vi "Kalibrationsprogramm_kapazitiv_yokogawaneu_2550.vi"(2 "Delay [ms]":u32=5000, 3 "Messzeit [ms]":u32=7000, 4 "B-Feld":dbl=5.0, 5 "error in (no error)":errorcluster, 6 "Startwert (V)":dbl=-5.0 min=-30.0 max=30.0 step=0.01, 7 "Stepsize (V)":dbl=1.0 min=0.0, 8 "Endwert (V)":dbl=4.0 min=-25.0 max=25.0 step=0.01) -> (15 "Ausgabe-Cluster":T1={" I (A)"=-5.009899999999962e-06, "Voltage"=42.05182, "B-Feld"=5.0, "Timestamp"=3396872323.6577854} {"Timestamp" format="%#_6f"}, 19 "error out":errorcluster)   [LabVIEW 2009]
uses:
  Instance           2 16Saved   Yokogawa .vi
  <vilib>/Utility/file.llb/Write To Spreadsheet File (DBL).vi
panel:
  out "XY Graph":cluster{dbl[], dbl[]}(graph)={[-5.004999999999957e-06, -3.989950000000041e-06, -2.990100500000007e-06, -1.999999999999981e-06, -9.9000000000001e-07, 2.2830184906463564e-22, 1.0000000000000002e-06, 2.0099999999999905e-06, 3.0000000000000013e-06, 4.009999999999992e-06, 5.00989999999996e-06, 3.999999999999972e-06, 2.9999999999999814e-06, 1.999999999999991e-06, 9.900000000000007e-07, -9.900000000000416e-09, -1.0000000000000023e-06, -2.0099999999999926e-06, -3.0000000000000035e-06, -4.009999999999994e-06, -5.009899999999962e-06], [40.83005555555556, 32.368543333333335, 24.101211666666668, 15.557882222222222, 7.205005, -1.09544, -9.418667777777777, -17.860119444444447, -26.364178888888894, -34.96848444444444, -43.319336666666665, -34.393308333333344, -25.663810555555553, -16.920877777777775, -8.246394444444444, 0.14445277777777776, 8.559738333333335, 17.03742388888889, 25.495266111111114, 33.88091111111111, 42.01979222222222]}
  in  "file path (dialog if empty)":path=path "D:/UserData/Matthias/Messungen/STO_LAOR103/110822/110822_R103_kalib_5T_0deg_1.txt"
  out "Done":bool=TRUE
  out "Data":bool
  out "UI":dbl=-5.009899999999962e-06
  out "Modus":string="F5SA"
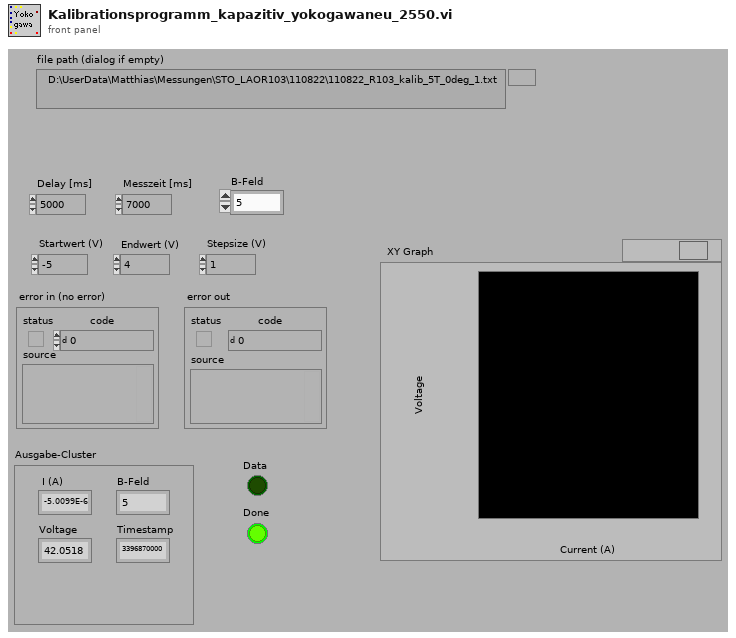
[diagram p1: front panel]
types:
  T1 = cluster{" I (A)":dbl, "Voltage":dbl, "B-Feld":dbl, "Timestamp":dbl}
  T2 = cluster{"UI":dbl, "capacitance":dbl, "B-Feld":dbl, dbl}
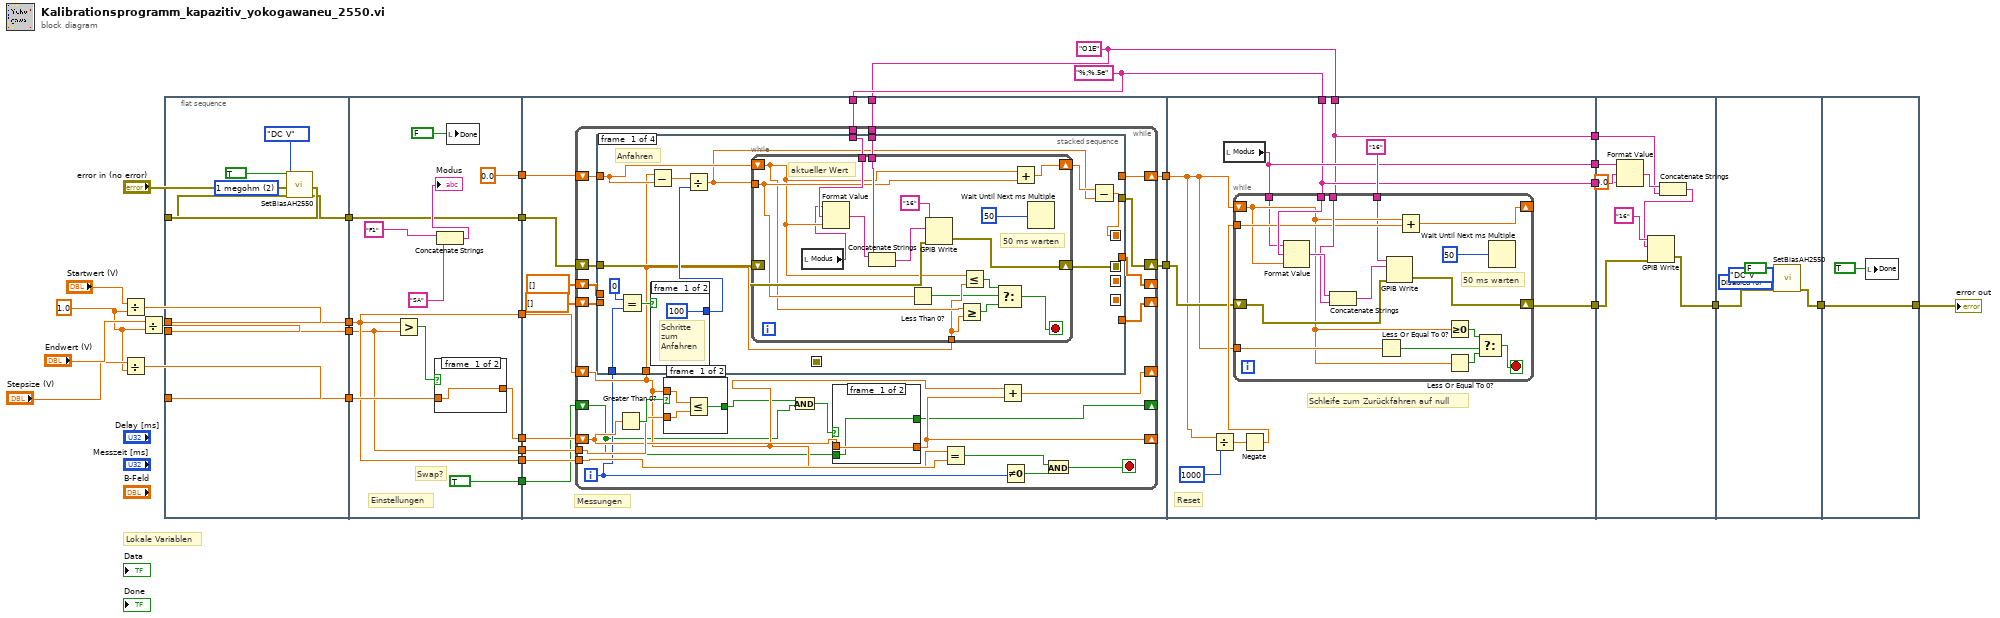
[diagram p0: block diagram]
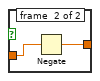
[diagram p2: hidden frame]
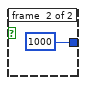
[diagram p3: hidden frame]
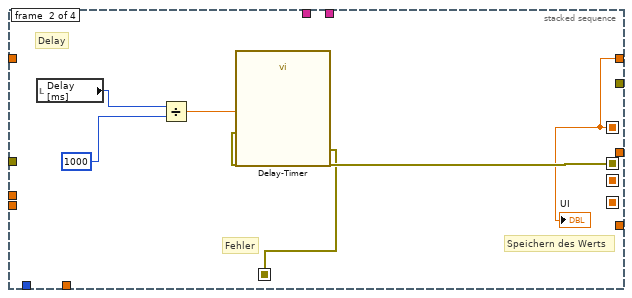
[diagram p4: hidden frame]
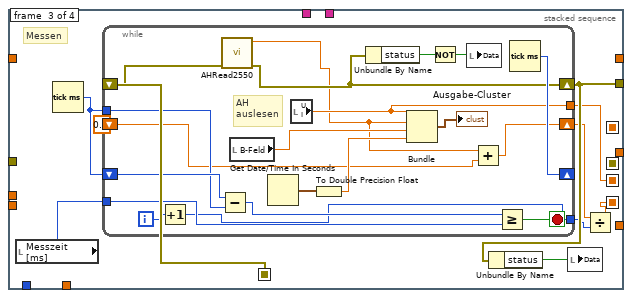
[diagram p5: hidden frame]
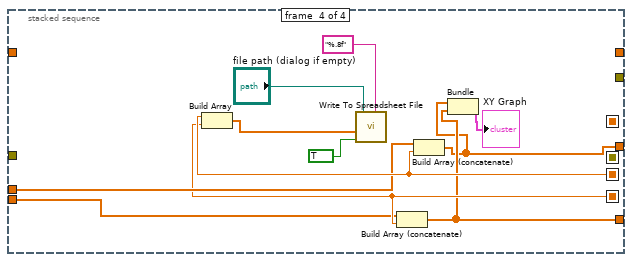
[diagram p6: hidden frame]
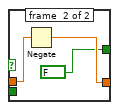
[diagram p7: hidden frame]
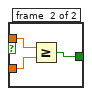
[diagram p8: hidden frame]
diagram:
  w7 = 1.0 ("y")
  w20 = "O1E"
  w21 = "%;%.5e"
  # "Lokale Variablen"
  n1 = Divide(x="Startwert (V)", y=w7) -> (x/y=w12:dbl)
  n2 = Divide(x="Stepsize (V)", y=w7) -> (x/y=w8:dbl)
  n3 = Divide(x="Endwert (V)", y=w7) -> (x/y=w10:dbl)
  n4 = flat-sequence {
    tunnel: "error in (no error)" -> [w34]
    tunnel: w8 -> [w36]
    tunnel: w10 -> [w37]
    tunnel: w12 -> [w38]
    tunnel: [w38] -> w6
    tunnel: [w37] -> w5
    tunnel: [w36] -> w4
    tunnel: [w33] -> w3
    tunnel: [w47] -> w30
    tunnel: [w48] -> w29
    tunnel: [w47] -> w28
    tunnel: [w46] -> w27
    tunnel: [0.0] -> w26
    tunnel: [w40] -> w25
    tunnel: [TRUE] -> w24
    tunnel: w6 -> [w47]
    tunnel: w5 -> [w46]
    tunnel: w4 -> [w49]
    tunnel: w3 -> [w40]
    tunnel: w30 -> [w66]
    tunnel: w29 -> [w64]
    tunnel: w28 -> [w65]
    tunnel: w27 -> [w63]
    tunnel: w26 -> [w62]
    tunnel: w21 -> [w61]
    tunnel: w20 -> [w60]
    tunnel: w25 -> [w59]
    tunnel: w24 -> [w57]
    tunnel: [w58] -> w23
    tunnel: [w56] -> w22
    tunnel: w23 -> [w189]
    tunnel: w22 -> [w187]
    tunnel: w21 -> [w184]
    tunnel: w20 -> [w183]
    tunnel: [w188] -> w18
    tunnel: [w185] -> w16
    tunnel: [w184] -> w15
    tunnel: [w183] -> w14
    tunnel: w18 -> [w217]
    tunnel: [w216] -> w2
    tunnel: w16 -> [w215]
    tunnel: w15 -> [w214]
    tunnel: w14 -> [w211]
    tunnel: w2 -> [w223]
    tunnel: [w222] -> w1
    tunnel: [w225] -> w19
    tunnel: w1 -> [w225]
    frame #0 {
      w31 = 2 items=["Disabled", "100 megohm", "1 megohm"] ("Bias (Off)")
      n5 = call "SetBiasAH2550.vi"("error in (no error)"=w34, "Bias (Off)"=w31, "V/A ?"=enum16{"DC V", "DC A"}."DC V", "On/Off"=TRUE) -> ("error out"=w33:errorcluster)  [unwired: 7 in]
    }
    frame #1 {
      # "Einstellungen"
      # "Swap?"
      n6 = Greater?(x=w47, y=w46) -> (0:w50:bool)
      n7 = case shown="False" w50 {
        tunnel: w49 -> [w51 w53]
        tunnel: [w51 w52] -> w48
        frame #0 {
        }
        frame #1 {
          n8 = Negate(x=w53) -> (-x=w52:dbl)
        }
      }
      n9 = Concatenate Strings("F1", "SA") -> (→"Modus":string)
      n10 = local write "Done"(FALSE) -> ()
    }
    frame #2 {
      # "Messungen"
      n11 = while {
        shift-right: [w80] -> _
        shift-left: w66 -> [w82]
        tunnel: w65 -> [w91]
        shift-right: [w81] -> _
        shift-left: w64 -> [w88]
        tunnel: w63 -> [w89]
        shift-right: [w83] -> w56
        shift-left: w62 -> [w87]
        tunnel: w61 -> [w86]
        tunnel: w60 -> [w85]
        shift-right: [w79] -> w58
        shift-left: w59 -> [w84]
        shift-right: [w74] -> _
        shift-left: w57 -> [w72]
        shift-right: [w69] -> _
        shift-left: dbl[] [] -> [w70]
        shift-right: [w68] -> _
        shift-left: dbl[] [] -> [w67]
        i -> [w78]
        stop <- w75 stop-if-true
        n12 = stacked-sequence {
          seq-local: [w97 _ _ _] -> [_ w130 _ _]
          seq-local: [_ w129 _ _] -> [_ _ w138 _]
          seq-local: [w92 _ _ _] -> [_ w125 _ _]
          seq-local: [_ _ w134 _] -> [_ _ _ w167]
          seq-local: [_ _ w131 _] -> [_ _ _ w165]
          tunnel: w78 -> [w104 _ _ _]
          tunnel: w87 -> [w96 _ _ _]
          tunnel: w82 -> [w95 _ _ _]
          tunnel: w86 -> [w100 _ _ _]
          tunnel: w85 -> [w99 _ _ _]
          tunnel: w84 -> [w98 _ _ _]
          tunnel: [_ w125 _ _] -> w83
          tunnel: [_ _ w137 _] -> w79
          tunnel: w70 -> [_ _ _ w166]
          tunnel: [_ _ _ w162] -> w69
          tunnel: [_ _ _ w163] -> w68
          tunnel: w67 -> [_ _ _ w164]
          frame #0 {
            # "Anfahren"
            n13 = Equal?(x=0, y=w104) -> (x = y?=w105:bool)
            n14 = Subtract(x=w95, y=w96) -> (x-y=w102:dbl)
            n15 = case shown="True" w105 {
              tunnel: [100 1000] -> w101
              frame #0 {
                # "Schritte\nzum\nAnfahren"
              }
              frame #1 {
              }
            }
            n16 = Divide(x=w102, y=w101) -> (x/y=w93:dbl)
            n17 = while {
              shift-right: [w122] -> w94
              shift-left: w96 -> [w113]
              tunnel: w95 -> [w112]
              tunnel: w93 -> [w114]
              tunnel: w100 -> [w121]
              tunnel: w99 -> [w119]
              shift-right: [w116] -> w97
              shift-left: w98 -> [w117]
              stop <- w108 stop-if-true
              # "50 ms warten"
              # "aktueller Wert"
              n18 = local read "Modus"() -> (w106:string)
              n19 = Format Value(string ("")=w106, format string=w121, value (0)=w113) -> (output string=w120:string)
              n20 = Concatenate Strings(w120, w119) -> (w118:string)
              n21 = Less Than 0?(x=w114) -> (x < 0?=w111:bool)
              n22 = GPIB Write(0:"16", 1:w118, 3:w117) -> (6:w116:errorcluster)  [unwired: 2 in, 1 out]
              n23 = Greater Or Equal?(x=w113, y=w112) -> (x >= y?=w109:bool)
              n24 = Less Or Equal?(x=w113, y=w112) -> (x <= y?=w110:bool)
              n25 = Select(t=w110, s=w111, f=w109) -> (s? t:f=w108:bool)
              n26 = Add(x=w113, y=w114) -> (x+y=w122:dbl)
              n27 = Wait Until Next ms Multiple(millisecond multiple=50) -> ()  [unwired: 1 out]
            }
            n28 = Subtract(x=w94, y=w93) -> (x-y=w92:dbl)
          }
          frame #1 {
            # "Delay"
            # "Speichern des Werts"
            # "Fehler"
            n29 = local read "Delay [ms]"() -> (w126:u32)
            n30 = Divide(x=w126, y=u32 1000) -> (x/y=w127:dbl)
            n31 = call "Delay-Timer"("error in (no error)"=w130, "Delay Time (s)"=w127) -> ("error out"=w129:errorcluster)  [unwired: 9 in]
            "UI" <- w125
          }
          frame #2 {
            # "Messen"
            n32 = local read "Messzeit [ms]"() -> (w139:u32)
            n33 = Tick Count (ms)() -> (millisecond timer value=w140:u32)
            n34 = while {
              shift-right: [w160] -> _
              shift-left: w140 -> [w159]
              tunnel: w140 -> [w158]
              tunnel: w139 -> [w156]
              shift-right: [w142] -> w137
              shift-left: w138 -> [w143]
              shift-right: [w148] -> w133
              shift-left: 0.0 -> [w147]
              tunnel: [w146] -> w134
              tunnel: [w144] -> w132
              i -> [w145]
              stop <- w157 stop-if-true
              # "AH\nauslesen"
              n35 = Increment(x=w145) -> (x+1=w144:i32)
              n36 = Subtract(x=w159, y=w158) -> (x-y=w155:u32)
              n37 = call "AHRead2550.vi"("error in (no error)"=w143) -> ("error out"=w142:errorcluster, "capacitance"=w141:dbl)  [unwired: 8 in, 1 out]
              n38 = local read "B-Feld"() -> (w153:dbl)
              n39 = Get Date/Time In Seconds() -> (seconds since 1Jan1904=w154:timestamp)
              n40 = local read "UI"() -> (w146:dbl)
              n41 = To Double Precision Float(number=w154) -> (double precision float=w152:dbl)
              n42 = Unbundle By Name(w142) -> ("status"=w151:bool)
              n43 = Bundle("UI"=w146, "capacitance"=w141, "B-Feld"=w153, w152) -> (→"Ausgabe-Cluster":T2)  [unwired: 1 in]
              n44 = Not(x=w151) -> (.not. x?=w150:bool)
              n45 = local write "Data"(w150) -> ()
              n46 = Add(x=w141, y=w147) -> (x+y=w148:dbl)
              n47 = Greater Or Equal?(x=w155, y=w156) -> (x >= y?=w157:bool)
              n48 = Tick Count (ms)() -> (millisecond timer value=w160:u32)
            }
            n49 = Unbundle By Name(w137) -> ("status"=w136:bool)
            n50 = local write "Data"(w136) -> ()
            n51 = Divide(x=w133, y=w132) -> (x/y=w131:dbl)
          }
          frame #3 {
            n52 = Build Array(w167, w165) -> (w171:dbl[])
            n53 = call-poly <vilib>:"Write To Spreadsheet File.vi"("format (%.3f)"="%.8f", "append to file? (new file:F)"=TRUE, "1D data"=w171, "file path (dialog if empty)"="file path (dialog if empty)") -> ()  [unwired: 4 in, 1 out]
            n54 = Build Array (concatenate)(w164, w165) -> (w163:dbl[])
            n55 = Build Array (concatenate)(w166, w167) -> (w162:dbl[])
            n56 = Bundle(w162, w163) -> (→"XY Graph":cluster{dbl[], dbl[]})  [unwired: 1 in]
          }
        }
        n57 = Greater Than 0?(x=w88) -> (x > 0?=w90:bool)
        n58 = case shown="True" w90 {
          tunnel: w89 -> [w178 w181]
          tunnel: w82 -> [w179 w182]
          tunnel: [w177 w180] -> w73
          frame #0 {
            n59 = Less Or Equal?(x=w179, y=w178) -> (x <= y?=w177:bool)
          }
          frame #1 {
            n60 = Greater Or Equal?(x=w182, y=w181) -> (x >= y?=w180:bool)
          }
        }
        n61 = And(x=w73, y=w72) -> (x .and. y?=w71:bool)
        n62 = case shown="False" w71 {
          tunnel: w88 -> [w173 w176]
          tunnel: [w173 w175] -> w81
          tunnel: [w172 FALSE] -> w74
          tunnel: w72 -> [w172 _]
          frame #0 {
          }
          frame #1 {
            n63 = Negate(x=w176) -> (-x=w175:dbl)
          }
        }
        n64 = Equal?(x=w82, y=w91) -> (x = y?=w77:bool)
        n65 = Add(x=w82, y=w81) -> (x+y=w80:dbl)
        n66 = Not Equal To 0?(x=w78) -> (x != 0?=w76:bool)
        n67 = And(x=w77, y=w76) -> (x .and. y?=w75:bool)
      }
    }
    frame #3 {
      # "Schleife zum Zurückfahren auf null"
      # "Reset"
      n68 = Divide(x=w187, y=1000) -> (x/y=w191:dbl)
      n69 = local read "Modus"() -> (w185:string)
      n70 = Negate(x=w191) -> (-x=w190:dbl)
      n71 = while {
        shift-right: [w199] -> _
        shift-left: w187 -> [w196]
        tunnel: w190 -> [w203]
        tunnel: w184 -> [w209]
        tunnel: w183 -> [w207]
        shift-right: [w197] -> w188
        shift-left: w189 -> [w205]
        tunnel: w187 -> [w198]
        tunnel: "16" -> [w195]
        tunnel: w185 -> [w194]
        stop <- w193 stop-if-true
        # "50 ms warten"
        n72 = Format Value(string ("")=w194, format string=w209, value (0)=w196) -> (output string=w208:string)
        n73 = Concatenate Strings(w208, w207) -> (w206:string)
        n74 = Less Or Equal To 0?(x=w198) -> (x <= 0?=w202:bool)
        n75 = GPIB Write(0:w195, 1:w206, 3:w205) -> (6:w197:errorcluster)  [unwired: 2 in, 1 out]
        n76 = Add(x=w196, y=w203) -> (x+y=w199:dbl)
        n77 = Greater Or Equal To 0?(x=w196) -> (x >= 0?=w201:bool)
        n78 = Less Or Equal To 0?(x=w196) -> (x <= 0?=w200:bool)
        n79 = Select(t=w201, s=w202, f=w200) -> (s? t:f=w193:bool)
        n80 = Wait Until Next ms Multiple(millisecond multiple=50) -> ()  [unwired: 1 out]
      }
    }
    frame #4 {
      n81 = Format Value(string ("")=w215, format string=w214, value (0)=0.0) -> (output string=w212:string)
      n82 = Concatenate Strings(w212, w211) -> (w210:string)
      n83 = GPIB Write(0:"16", 1:w210, 3:w217) -> (6:w216:errorcluster)  [unwired: 2 in, 1 out]
    }
    frame #5 {
      w219 = 0 items=["Disabled", "100 megohm", "1 megohm"] ("Bias (Off)")
      n84 = call "SetBiasAH2550.vi"("error in (no error)"=w223, "Bias (Off)"=w219, "V/A ?"=enum16{"DC V", "DC A"}."DC V", "On/Off"=FALSE) -> ("error out"=w222:errorcluster)  [unwired: 7 in]
    }
    frame #6 {
      n85 = local write "Done"(TRUE) -> ()
    }
  }
  "error out" <- w19
